vi "Execute.vi"(10 "Msg":refnum<class "Msg.lvclass">, 11 "Actor in":refnum<class "Actor.lvclass">) -> (3 "Actor out":refnum<class "Actor.lvclass">)   [LabVIEW 2021, in "jettl.lvlib" / "Actor.lvlib" / "Actor.lvclass"]
uses:
  Actor.lvclass
  Msg/Msg.lvclass
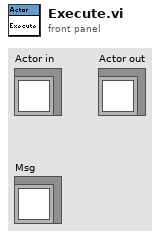
[diagram p1: front panel]
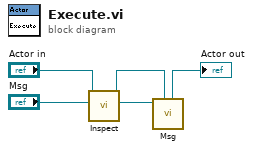
[diagram p0: block diagram]
diagram:
  n1 = call-dynamic "Inspect.vi"("Msg in"="Msg", "Actor in"="Actor in") -> ("Msg out"=w3:refnum<class "Msg.lvclass">, "Actor out"=w2:refnum<class "Actor.lvclass">)  [unwired: 8 in]
  n2 = call-dynamic "Msg.vi"("Actor in"=w2, "Msg in"=w3) -> ("Actor out"=→"Actor out":refnum<class "Actor.lvclass">)  [unwired: 9 in]
